vi "_Convert Center Width.vi"(4 "Center/Width":bool, 5 "Run Mode":T1, 6 "StepMass Changed":bool, 7 "Step Mass":dbl, 8 "Stop Mass":dbl, 9 "Start Mass":dbl) -> (1 "Step Mass (amu)":dbl, 2 "Stop Mass (amu)":dbl, 3 "Start Mass (amu)":dbl)   [LabVIEW 2012]
uses:
  Type/_Run Mode.ctl
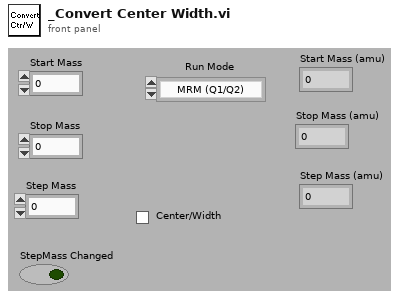
[diagram p1: front panel]
types:
  T1 = typedef "_Run Mode.ctl" = enum16{"MRM (Q1/Q2)", "Q1 Scan", "Q1 SRM", "Q2 Scan", "Q2 SRM", "Product Scan", "Precursor Scan", "Neutral Loss", "Neutral Gain"}
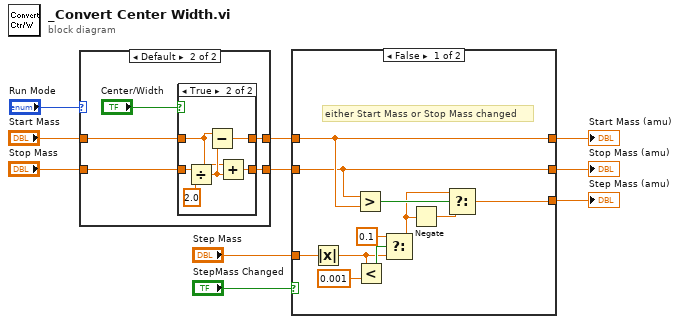
[diagram p0: block diagram]
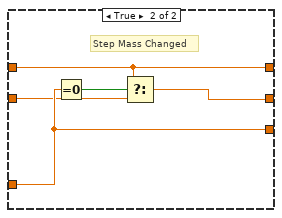
[diagram p4: hidden frame]
diagram:
  n1 = case shown="Default" "Run Mode" {
    tunnel: "Start Mass" -> [w12 w16]
    tunnel: "Stop Mass" -> [w11 w15]
    tunnel: [w12 w14] -> w3
    tunnel: [w11 w13] -> w2
    frame "MRM (Q1/Q2)", "Q1 SRM", "Q2 SRM" {
    }
    frame Default {
      n2 = case shown="True" "Center/Width" {
        tunnel: w16 -> [w19 w20]
        tunnel: w15 -> [w18 w25]
        tunnel: [w19 w22] -> w14
        tunnel: [w18 w23] -> w13
        frame False {
        }
        frame True {
          n3 = Divide(x=w25, y=2.0) -> (x/y=w21:dbl)
          n4 = Subtract(x=w20, y=w21) -> (x-y=w22:dbl)
          n5 = Add(x=w20, y=w21) -> (x+y=w23:dbl)
        }
      }
    }
  }
  n6 = case shown="False" "StepMass Changed" {
    tunnel: [w27 w38] -> w9
    tunnel: w3 -> [w27 w38]
    tunnel: [w26 w40] -> w8
    tunnel: w2 -> [w26 w39]
    tunnel: "Step Mass" -> [w36 w41]
    tunnel: [w35 w41] -> w7
    frame False {
      # "either Start Mass or Stop Mass changed"
      n7 = Absolute Value(x=w36) -> (abs(x)=w30:dbl)
      n8 = Greater?(x=w26, y=w27) -> (0:w34:bool)
      n9 = Less?(x=w30, y=0.001) -> (x < y?=w31:bool)
      n10 = Select(t=0.1, s=w31, f=w30) -> (s? t:f=w28:dbl)
      n11 = Negate(x=w28) -> (-x=w33:dbl)
      n12 = Select(t=w28, s=w34, f=w33) -> (s? t:f=w35:dbl)
    }
    frame True {
      # "Step Mass Changed"
      n13 = Equal To 0?(x=w41) -> (x = 0?=w37:bool)
      n14 = Select(t=w38, s=w37, f=w39) -> (s? t:f=w40:dbl)
    }
  }
  "Start Mass (amu)" <- w9
  "Stop Mass (amu)" <- w8
  "Step Mass (amu)" <- w7
